vi "Q.Enqueue Error_Warning.vi"(5 "Top of Q(T)":bool=TRUE, 7 "Q Name":string, 8 "Error In":errorcluster, 9 "Error/Warning":errorcluster, 10 "Warning(F)/Error(T)":bool=TRUE, 11 "Q In":refnum<queue>) -> (0 "error out":errorcluster, 3 "Q Out":refnum<queue>)   [LabVIEW 2024, in "EQMF.lvlib" / "Queue Utils.lvlib"]
doc: "This VI enqueues the EXIT command.\n Queue element 'Cmd' = \"Exit\"\n\nThis VI obtains the queue by name or by queue reference.\nIf the 'Q Name' input is empty then it obtains the queue by the 'Q In\" reference.\nIf the 'Q Name' input is NOT empty then it obtains the queue by the this name.\n If a queue is ontained by name and the queue does not already exits, an error is generated.\n\nThe 'Top of Q' input is TRUE by default.\nThis input will cause this item to be enqueued on the top of the queue when it is TRUE.\n\nThe 'Flush Q' input is FALSE by default.\nThis input will cause the queue to be flushed when it is TRUE."
uses:
  Queue Utils.lvlib
  Q.Element.ctl
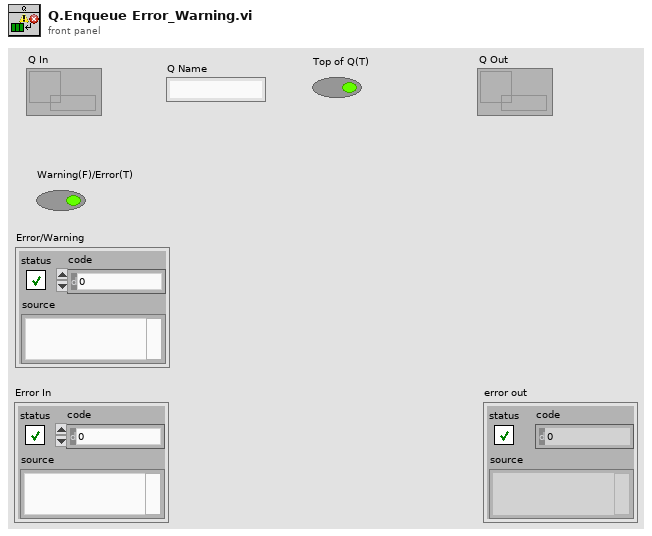
[diagram p1: front panel]
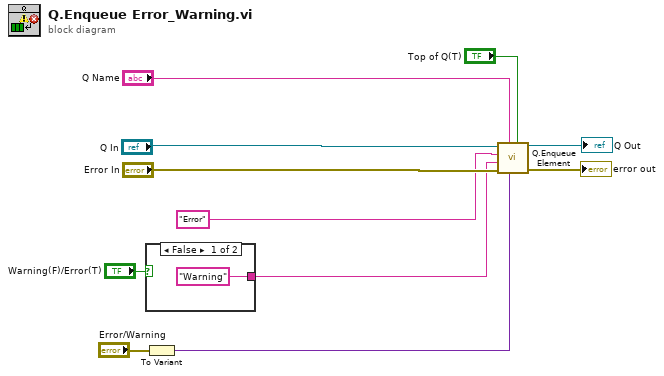
[diagram p0: block diagram]
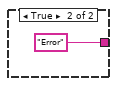
[diagram p2: hidden frame]
diagram:
  n1 = case shown="False" "Warning(F)/Error(T)" {
    tunnel: ["Warning" ("Cmd") "Error" ("Cmd")] -> w1
    frame False {
    }
    frame True {
    }
  }
  n2 = To Variant(anything="Error/Warning") -> (Variant=w4:variant)
  n3 = call "Q.Enqueue Element.vi"("Top of Q"="Top of Q(T)", "Data1"=w4, "Q Name"="Q Name", "error in"="Error In", "Sub"=w1, "Cmd"="Error", "Q In"="Q In") -> ("error out"=→"error out":errorcluster, "Q Out"=→"Q Out":refnum<queue>)  [unwired: 3 in]
